vi "Scale Cell Temp.vi"(11 "Numeric in":u8) -> (3 "Numeric out":dbl)   [LabVIEW 2015]
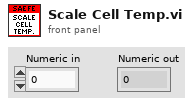
[diagram p1: front panel]
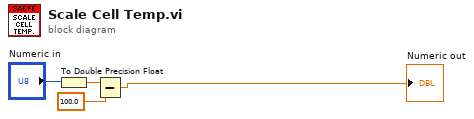
[diagram p0: block diagram]
diagram:
  n1 = To Double Precision Float(number="Numeric in") -> (double precision float=w2:dbl)
  n2 = Subtract(x=w2, y=100.0) -> (x-y=→"Numeric out":dbl)
